vi "AVI-Get all split file paths.vi"(8 "error in (no error)":errorcluster, 11 "AVI2 video Path":path) -> (0 "error out":errorcluster, 3 "Split AVI files path&name":path[](array[path]))   [LabVIEW 2020]
panel:
  # "<--- Can be any of a series of split files"
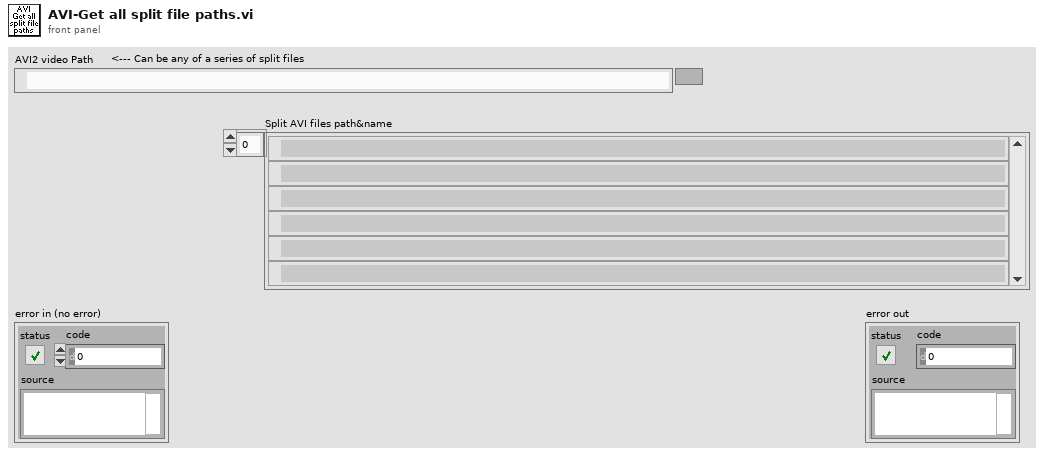
[diagram p1: front panel]
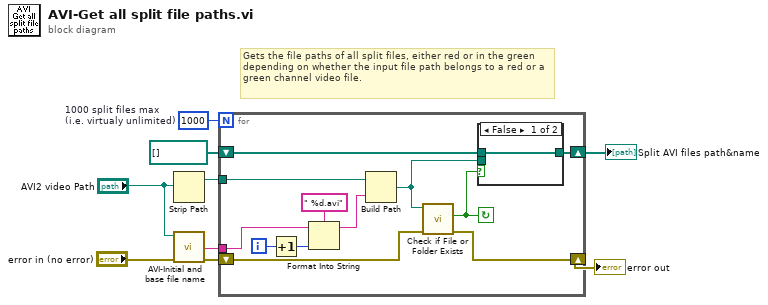
[diagram p0: block diagram]
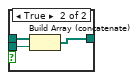
[diagram p2: hidden frame]
diagram:
  w4 = 1000  # 1000 split files max (i.e. virtualy unlimited)
  # "Gets the file paths of all split files, either red or in the green depending on whether the input file path belongs to a red or a green channel video file."
  n1 = Strip Path(path="AVI2 video Path") -> (stripped path=w2:path)  [unwired: 1 out]
  n2 = call "AVI-Initial and base file name.vi"("error in (no error)"="error in (no error)", "AVI file path & name"="AVI2 video Path") -> ("error out"=w8:errorcluster, "Base file name"=w5:string)  [unwired: 5 in, 3 out]
  n3 = for {
    N: w4 -> [_]
    tunnel: w2 -> [w18]
    tunnel: w5 -> [w17]
    shift-right: [w14] -> w3
    shift-left: path[] [] -> [w13]
    shift-right: [w11] -> w9
    shift-left: w8 -> [w10]
    i -> [w20]
    stop <- w12 continue-if-true
    n4 = Increment(x=w20) -> (x+1=w16:i32)
    n5 = Format Into String(format string=" %d.avi", initial string=w17, w16) -> (resulting string=w19:string)  [unwired: 1 in, 1 out]
    n6 = Build Path(base path=w18, name or relative path=w19) -> (appended path=w15:path)
    n7 = call <vilib>:"Check if File or Folder Exists.vi"("error in (no error)"=w10, "path"=w15) -> ("error out"=w11:errorcluster, "file or folder exists?"=w12:bool)  [unwired: 7 in, 1 out]
    n8 = case shown="False" w12 {
      tunnel: w15 -> [_ w25]
      tunnel: [w22 w24] -> w14
      tunnel: w13 -> [w22 w23]
      frame False {
      }
      frame True {
        n9 = Build Array (concatenate)(w23, w25) -> (w24:path[])
      }
    }
  }
  "Split AVI files path&name" <- w3
  "error out" <- w9
